vi "VI Tree.vi"   [LabVIEW 2013]
doc: "This is the instrument driver for the <INSTRUMENT NAME>. The VI Tree displays all the user-callable VIs of the instrument driver in an organized table."
uses:
  <instrlib>/ZBOX_IS/ZBOX_IS.lvlib
panel:
  # "(c) 2007 <Enter Company Name Here>.  ALL RIGHTS RESERVED."
  # "SEE DIAGRAM\nFOR VI TREE."
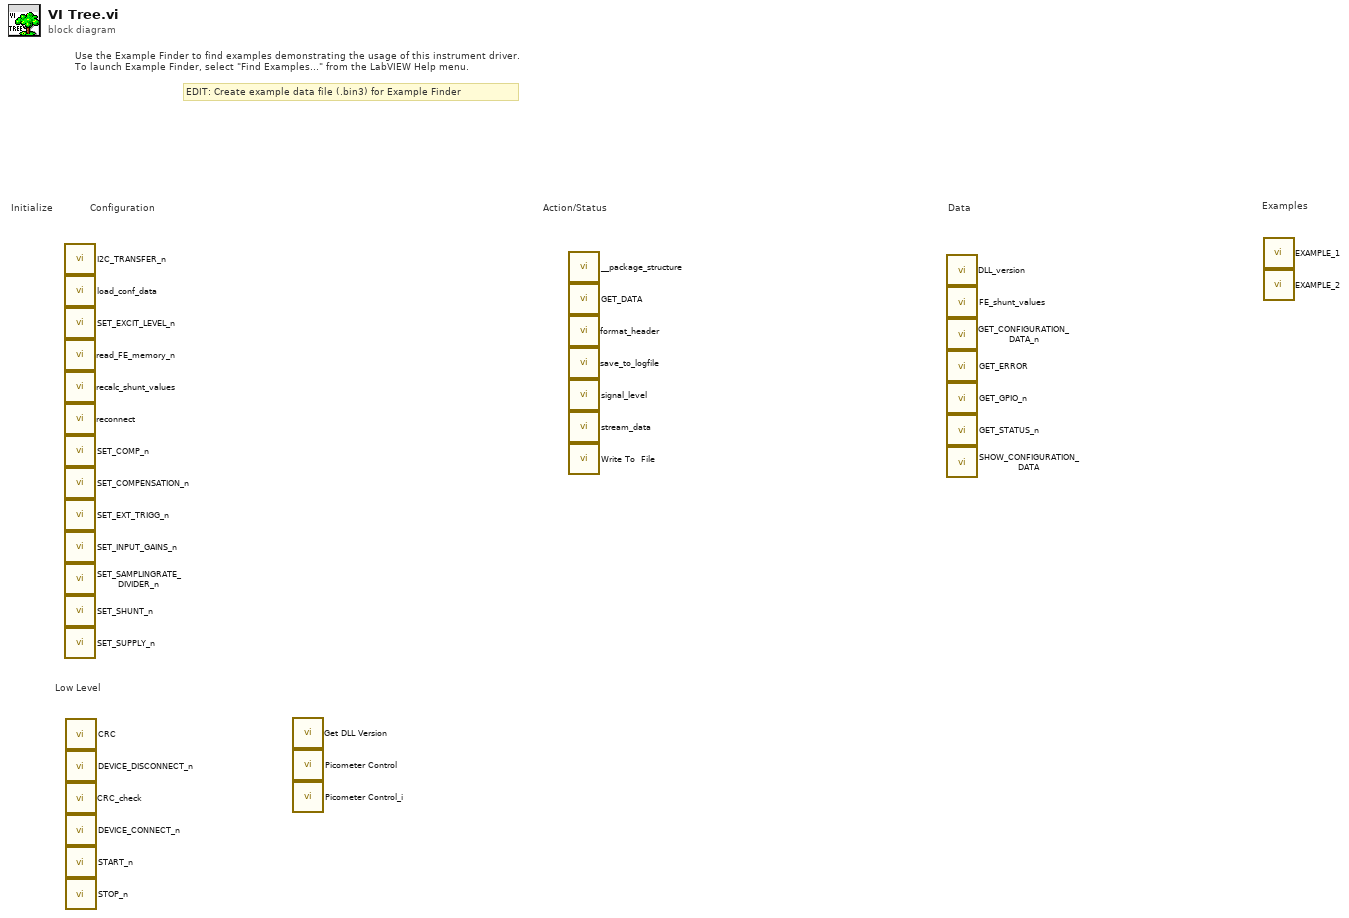
[diagram p0: block diagram]
diagram:
  # "Low Level"
  # "Examples"
  # "EDIT: Create example data file (.bin3) for Example Finder"
  # "Use the Example Finder to find examples demonstrating the usage of this instrument driver.\nTo launch Example Finder, select \"Find Examples...\" from the LabVIEW Help menu."
  # "Configuration"
  # "Data"
  # "Action/Status"
  # "Initialize"
  n1 = call <instrlib>:"I2C_TRANSFER_n.vi"() -> ()  [unwired: 11 in, 5 out]
  n2 = call <instrlib>:"load_conf_data.vi"() -> ()  [unwired: 14 in, 2 out]
  n3 = call <instrlib>:"SET_EXCIT_LEVEL_n.vi"() -> ()  [unwired: 14 in, 2 out]
  n4 = call <instrlib>:"read_FE_memory_n.vi"() -> ()  [unwired: 11 in, 5 out]
  n5 = call <instrlib>:"recalc_shunt_values.vi"() -> ()  [unwired: 16 in, 4 out]
  n6 = call <instrlib>:"reconnect.vi"() -> ()  [unwired: 13 in, 3 out]
  n7 = call <instrlib>:"SET_COMP_n.vi"() -> ()  [unwired: 14 in, 2 out]
  n8 = call <instrlib>:"SET_COMPENSATION_n.vi"() -> ()  [unwired: 14 in, 2 out]
  n9 = call <instrlib>:"SET_EXT_TRIGG_n.vi"() -> ()  [unwired: 14 in, 2 out]
  n10 = call <instrlib>:"SET_INPUT_GAINS_n.vi"() -> ()  [unwired: 14 in, 2 out]
  n11 = call <instrlib>:"SET_SAMPLINGRATE_DIVIDER_n.vi"() -> ()  [unwired: 14 in, 2 out]
  n12 = call <instrlib>:"SET_SHUNT_n.vi"() -> ()  [unwired: 14 in, 2 out]
  n13 = call <instrlib>:"SET_SUPPLY_n.vi"() -> ()  [unwired: 14 in, 2 out]
  n14 = call <instrlib>:"CRC.vi"() -> ()  [unwired: 9 in, 3 out]
  n15 = call <instrlib>:"DEVICE_DISCONNECT_n.vi"() -> ()  [unwired: 14 in, 2 out]
  n16 = call <instrlib>:"CRC_check.vi"() -> ()  [unwired: 11 in, 5 out]
  n17 = call <instrlib>:"DEVICE_CONNECT_n.vi"() -> ()  [unwired: 12 in, 4 out]
  n18 = call <instrlib>:"START_n.vi"() -> ()  [unwired: 14 in, 2 out]
  n19 = call <instrlib>:"STOP_n.vi"() -> ()  [unwired: 14 in, 2 out]
  n20 = call <instrlib>:"Get DLL Version.vi"() -> ()  [unwired: 9 in, 3 out]
  n21 = call <instrlib>:"Picometer Control.vi"() -> ()  [unwired: 11 in, 5 out]
  n22 = call <instrlib>:"Picometer Control_i.vi"() -> ()  [unwired: 11 in, 5 out]
  n23 = call <instrlib>:"__package_structure.vi"() -> ()  [unwired: 9 in, 11 out]
  n24 = call <instrlib>:"GET_DATA.vi"() -> ()  [unwired: 13 in, 3 out]
  n25 = call <instrlib>:"format_header.vi"() -> ()  [unwired: 15 in, 1 out]
  n26 = call <instrlib>:"save_to_logfile.vi"() -> ()  [unwired: 18 in, 2 out]
  n27 = call <instrlib>:"signal_level.vi"() -> ()  [unwired: 15 in, 1 out]
  n28 = call <instrlib>:"stream_data.vi"() -> ()  [unwired: 15 in, 1 out]
  n29 = call <instrlib>:"Write To  File.vi"() -> ()  [unwired: 8 in, 1 out]
  n30 = call <instrlib>:"DLL_version.vi"() -> ()  [unwired: 13 in, 3 out]
  n31 = call <instrlib>:"FE_shunt_values.vi"() -> ()  [unwired: 16 in, 4 out]
  n32 = call <instrlib>:"GET_CONFIGURATION_DATA_n.vi"() -> ()  [unwired: 9 in, 11 out]
  n33 = call <instrlib>:"GET_ERROR.vi"() -> ()  [unwired: 13 in, 3 out]
  n34 = call <instrlib>:"GET_GPIO_n.vi"() -> ()  [unwired: 13 in, 3 out]
  n35 = call <instrlib>:"GET_STATUS_n.vi"() -> ()  [unwired: 12 in, 4 out]
  n36 = call <instrlib>:"SHOW_CONFIGURATION_DATA.vi"() -> ()  [unwired: 11 in, 1 out]
  n37 = call <instrlib>:"EXAMPLE_1.vi"() -> ()  [unwired: 1 in]
  n38 = call <instrlib>:"EXAMPLE_2.vi"() -> ()  [unwired: 12 in]
